vi "test_objectScalar.vi"(8 "error in (no error)":errorcluster) -> (0 "error out":errorcluster)   [LabVIEW 2013]
uses:
  test-TestableClass/Caraya-TestableClass.lvclass
  test-TestableClass/Caraya-TestableClass.lvclass/Caraya-TestableClass.ctl
  run-tests/Run Test (Object).vi
  Caraya.lvlib
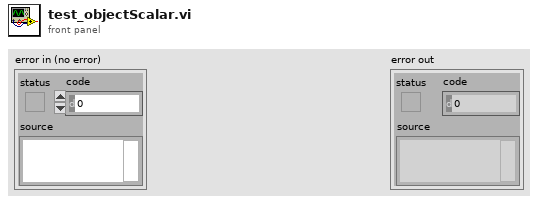
[diagram p1: front panel]
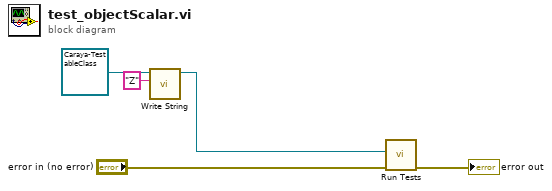
[diagram p0: block diagram]
diagram:
  n1 = call "Write String.vi"("String"="Z", "Caraya-TestableClass in"=refnum<class "Caraya-TestableClass.lvclass"> refnum ("Caraya-TestableClass.lvclass")) -> ("Caraya-TestableClass out"=w2:refnum<class "Caraya-TestableClass.lvclass">)  [unwired: 9 in]
  n2 = call-poly "Run Tests.vi"("error in"="error in (no error)", "Object"=w2) -> ("error out"=→"error out":errorcluster)  [unwired: 9 in]
